vi "Export.vi"() -> ()   [LabVIEW 2018, in "Scripts.lvlib"]
uses:
  Scripts.lvlib
  <vilib>/Field R&D Services/Labricator/Toolkit/Type Definitions/LabVIEW Versions.ctl
  <vilib>/Field R&D Services/Labricator/Toolkit/Support/Find Target Project Root.vi
  <vilib>/Field R&D Services/Labricator/Toolkit/File Constants/Source Directory.vi
  <vilib>/Field R&D Services/Labricator/Toolkit/File Constants/Target Directory.vi
  <vilib>/Field R&D Services/Labricator/Toolkit/File Constants/Project File.vi
  <vilib>/Field R&D Services/Labricator/Toolkit/Support/Project Save for Previous.vi
  <vilib>/Utility/libraryn.llb/Recursive File List.vi
  <vilib>/Utility/libraryn.llb/Get File Extension.vi
  <vilib>/Utility/error.llb/Error Cluster From Error Code.vi
  <vilib>/Field R&D Services/Labricator/Toolkit/Support/Copy Help.vi
  <vilib>/Field R&D Services/Labricator/Toolkit/Field_RnD_Services_Labricator_Toolkit.lvlib
panel:
  in  "Copy Help? (T)":bool=TRUE
  in  "LabVIEW Previous Version":T1
  # "Overview: Saves the project in a previous version of LabVIEW\nRequirements: Labricator Development Kit\nInstructions: Run this VI.\n\nThis VI attempts to automate saving the entire project in a previous version of LabVIEW. This is the first step in creating a VIP, but sometimes it is necessary to just export the source code in an earlier version. This VI automates the following manual steps:\n\n1. Save the current project for LabVIEW 2009\n    a. From the Project Explorer window, select File>>Save for Previous Version... A new dialog will appear.\n    b. Select 9.0 from the drop down menu.\n    c. Click Save.... A new dialog will appear. Create a \"target\\9.0\" folder hierarchy in the root project folder (same location as the project file,    \n        .lvproj) if it does not already exist.\n    d. Click OK. All of the contents of the project will be saved to LabVIEW 2009."
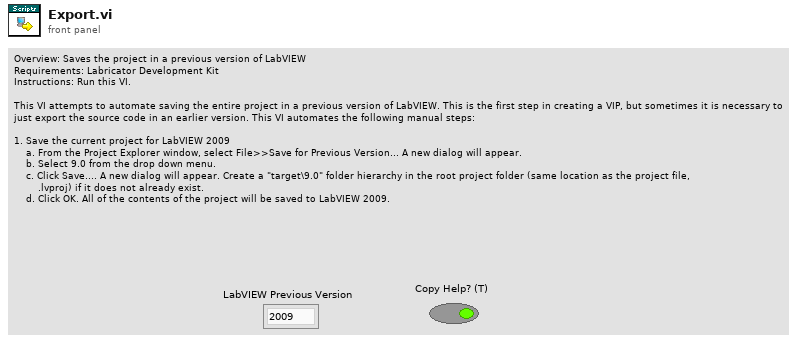
[diagram p1: front panel]
types:
  T1 = typedef "Field_RnD_Services_Labricator_Toolkit.lvlib/LabVIEW Versions.ctl" = enum16{"2009", "2010", "2011", "2012", "2013", "2014", "2015", "2016", "2017", "2018"}
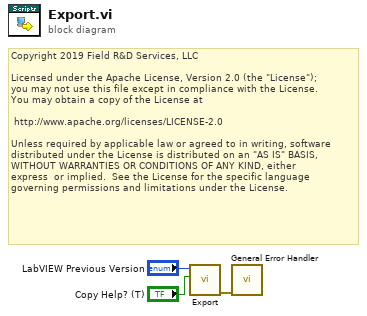
[diagram p0: block diagram]
diagram:
  # "Copyright 2019 Field R&D Services, LLC\n\nLicensed under the Apache License, Version 2.0 (the \"License\");\nyou may not use this file except in compliance with the License.\nYou may obtain a copy of the License at\n\n\thttp://www.apache.org/licenses/LICENSE-2.0\n\nUnless required by applicable law or agreed to in writing, software\ndistributed under the License is distributed on an \"AS IS\" BASIS,\nWITHOUT WARRANTIES OR CONDITIONS OF ANY KIND, either \nexpress  or implied.  See the License for the specific language \ngoverning permissions and limitations under the License."
  n1 = call <vilib>:"Export.vi"("Copy Help? (T)"="Copy Help? (T)", "LabVIEW Previous Version"="LabVIEW Previous Version") -> ("Error Out"=w2:errorcluster)  [unwired: 9 in]
  n2 = call <vilib>:"General Error Handler.vi"("error in (no error)"=w2) -> ()  [unwired: 10 in, 5 out]
